vi "mtg reader - update cursor position.vi"(9 "Coords":T1, 10 "time at cursor":refnum<vi>, 11 "WaveformChart in":refnum<vi>) -> ()   [LabVIEW 2025]
uses:
  <vilib>/Utility/miscctls.llb/LVPoint32TypeDef.ctl
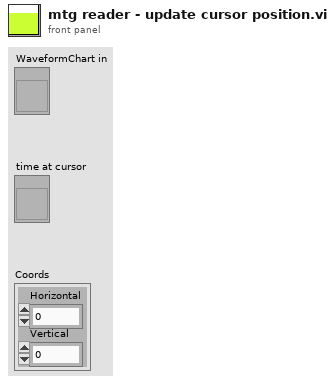
[diagram p1: front panel]
types:
  T1 = typedef "LVPoint32TypeDef.ctl" = cluster{"Horizontal":i32, "Vertical":i32}
  T2 = typedef "LVRectTypeDef.ctl" = cluster{"Left":i16, "Top":i16, "Right":i16, "Bottom":i16}
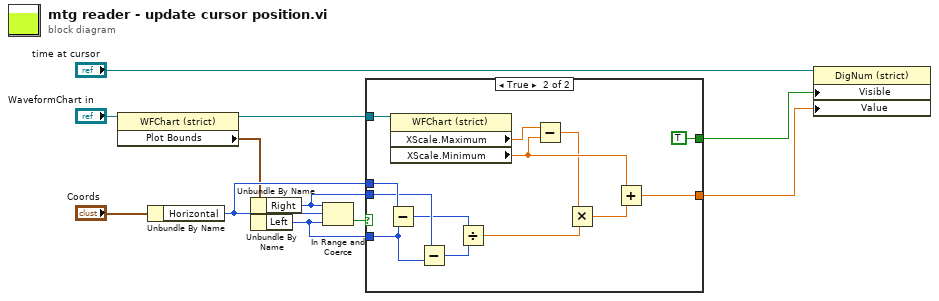
[diagram p0: block diagram]
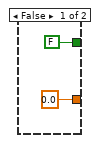
[diagram p2: hidden frame]
diagram:
  n1 = property class="WFChart (strict)"(reference="WaveformChart in") -> (reference out=w1:refnum<vi>, "Plot Bounds"=w7:T2)  [unwired: 1 in, 1 out]
  n2 = Unbundle By Name("Coords") -> ("Horizontal"=w11:i32)
  n3 = Unbundle By Name(w7) -> ("Right"=w9:i16)
  n4 = Unbundle By Name(w7) -> ("Left"=w10:i16)
  n5 = In Range and Coerce(upper limit=w9, x=w11, lower limit=w10) -> (In Range?=w8:bool)  [unwired: 1 out]
  n6 = case shown="True" w8 {
    tunnel: w9 -> [_ w25]
    tunnel: w10 -> [_ w24]
    tunnel: w11 -> [_ w26]
    tunnel: [0.0 w19] -> w3
    tunnel: [FALSE TRUE] -> w2
    tunnel: w1 -> [_ w17]
    frame False {
    }
    frame True {
      n7 = Subtract(x=w26, y=w24) -> (x-y=w22:i32)
      n8 = property class="WFChart (strict)"(reference=w17) -> ("XScale.Maximum"=w16:dbl, "XScale.Minimum"=w15:dbl)  [unwired: 1 in, 2 out]
      n9 = Subtract(x=w25, y=w24) -> (x-y=w23:i16)
      n10 = Divide(x=w22, y=w23) -> (x/y=w21:dbl)
      n11 = Subtract(x=w16, y=w15) -> (x-y=w14:dbl)
      n12 = Multiply(x=w14, y=w21) -> (x*y=w20:dbl)
      n13 = Add(x=w15, y=w20) -> (x+y=w19:dbl)
    }
  }
  n14 = property class="DigNum (strict)"(reference="time at cursor", "Visible"=w2, "Value"=w3) -> ()  [unwired: 1 in, 2 out]
